vi "vectorsTurningAround.vi"(0 "KickToSkill in":refnum<class "KickToSkill.lvclass">, 5 "Game":refnum<class "Game.lvclass">, 7 "Target":dbl[](array[numeric]), 9 "Robot in":refnum<class "Robot.lvclass">, 11 "error in (no error)":errorcluster) -> (1 "Robot - Target":dbl[](array[numeric]) format="%0.2f", 3 "Ball - Target":dbl[](array[numeric]) format="%0.2f", 4 "KickToSkill out":refnum<class "KickToSkill.lvclass">, 6 "Robot - Ball norm":dbl format="%0.2f", 10 "Robot - Target norm":dbl format="%0.2f", 12 "Ball - Target norm":dbl format="%0.2f", 14 "Robot - Ball":dbl[](array[numeric]) format="%0.2f", 15 "error out":errorcluster)   [LabVIEW 2021, in "KickToSkill.lvclass"]
uses:
  KickToSkill.lvclass
  Game_class/Game.lvclass
  Robot_class/Robot.lvclass
  D:/RoboIme/horie/SSL_AI/Object_class/Object.lvclass
  Game_class/Game.lvclass/Game.ctl
  Object_class/Object.lvclass/Object.ctl
  <vilib>/Analysis/baseanly.llb/Unit Vector (DBL).vi
  Object_class/Read position(x,y).vi
  Game_class/Read BallRef.vi
  Ball_class/Ball.lvclass
  <vilib>/Analysis/NI_AALBase.lvlib
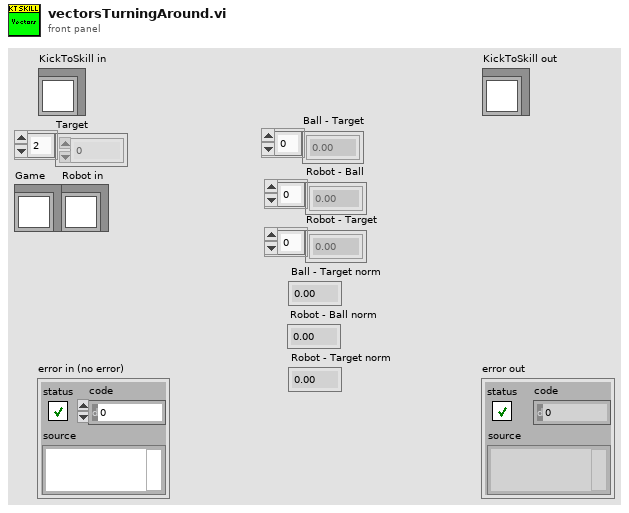
[diagram p1: front panel]
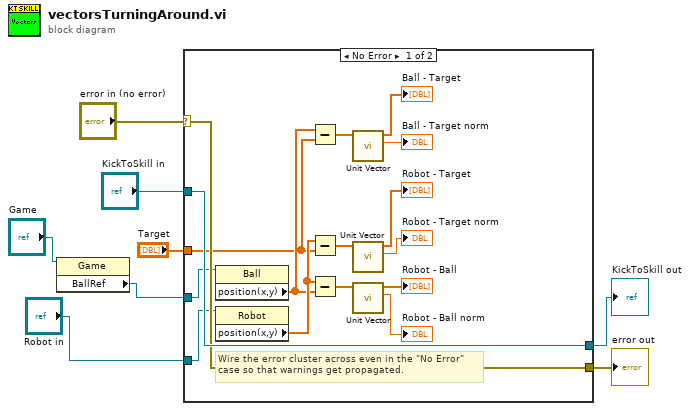
[diagram p0: block diagram]
diagram:
  n1 = property class="Game"(reference="Game") -> ("BallRef"=w1:refnum<class "Ball.lvclass">)  [unwired: 1 in, 2 out]
  n2 = case shown="No Error" "error in (no error)" {
    selector: "error in (no error)" -> [w23 w26]
    tunnel: [w23 w26] -> w7
    tunnel: [w24 w25] -> w5
    tunnel: "KickToSkill in" -> [w24 w25]
    tunnel: "Robot in" -> [w18 _]
    tunnel: w1 -> [w19 _]
    tunnel: "Target" -> [w20 _]
    frame No Error {
      # "Wire the error cluster across even in the \"No Error\"\ncase so that warnings get propagated."
      n3 = property class="Ball"(reference=w19) -> ("position(x,y)"=w21:dbl[])  [unwired: 1 in, 2 out]
      n4 = property class="Robot"(reference=w18) -> ("position(x,y)"=w22:dbl[])  [unwired: 1 in, 2 out]
      n5 = Subtract(x=w21, y=w20) -> (x-y=w15:dbl[])
      n6 = Subtract(x=w22, y=w20) -> (x-y=w16:dbl[])
      n7 = Subtract(x=w22, y=w21) -> (x-y=w17:dbl[])
      n8 = call-poly <vilib>:"Unit Vector.vi"("Input Vector"=w15) -> ("norm"=→"Ball - Target norm":dbl, "Unit Vector"=→"Ball - Target":dbl[])  [unwired: 8 in, 1 out]
      n9 = call-poly <vilib>:"Unit Vector.vi"("Input Vector"=w16) -> ("norm"=→"Robot - Target norm":dbl, "Unit Vector"=→"Robot - Target":dbl[])  [unwired: 8 in, 1 out]
      n10 = call-poly <vilib>:"Unit Vector.vi"("Input Vector"=w17) -> ("norm"=→"Robot - Ball norm":dbl, "Unit Vector"=→"Robot - Ball":dbl[])  [unwired: 8 in, 1 out]
    }
    frame Error {
    }
  }
  "error out" <- w7
  "KickToSkill out" <- w5
